vi "Write Timeout.vi"(8 "error in (no error)":errorcluster, 10 "Timeout":i32, 11 "BaseMessage in":refnum<class "BaseMessage.lvclass">) -> (0 "error out":errorcluster, 3 "BaseMessage out":refnum<class "BaseMessage.lvclass">)   [LabVIEW 2013, in "BaseMessage.lvclass"]
doc: "Time to wait before generating a timeout error if no response arrives for this message. A value of 0 means do not wait at all for a response, and a negative value means wait forever"
uses:
  BaseMessage.lvclass
  BaseMessage.lvclass/BaseMessage.ctl
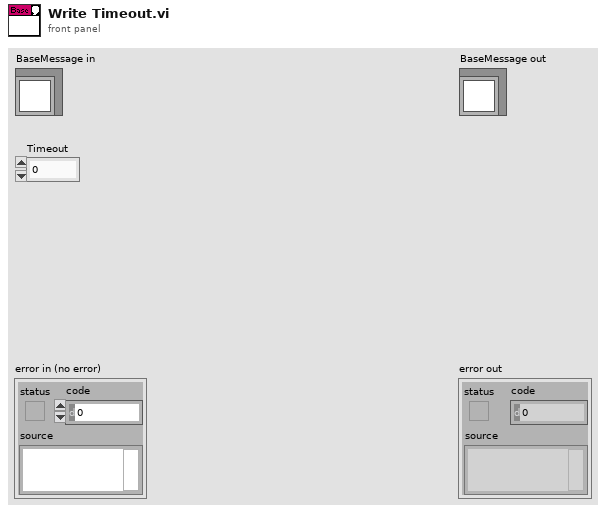
[diagram p1: front panel]
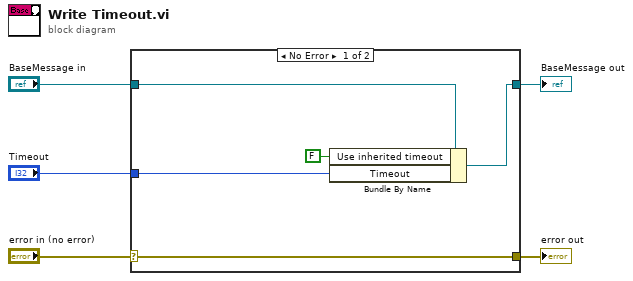
[diagram p0: block diagram]
diagram:
  n1 = case shown="No Error" "error in (no error)" {
    selector: "error in (no error)" -> [w10 w11]
    tunnel: [w10 w11] -> w4
    tunnel: [w9 w12] -> w2
    tunnel: "BaseMessage in" -> [w7 w12]
    tunnel: "Timeout" -> [w8 _]
    frame No Error {
      n2 = Bundle By Name(cluster=w7, "Use inherited timeout"=FALSE, "Timeout"=w8) -> (w9:refnum<class "BaseMessage.lvclass">)
    }
    frame Error {
    }
  }
  "error out" <- w4
  "BaseMessage out" <- w2
